vi "set_context.vi"(8 "error in (no error)":errorcluster, 9 "remote address":string, 10 "remote port":u16, 11 "WebSocket Queue Logger in":refnum<class "WebSocket Queue Logger.lvclass">) -> (0 "error out":errorcluster, 3 "WebSocket Queue Logger out":refnum<class "WebSocket Queue Logger.lvclass">)   [LabVIEW 2019, in "WebSocket Server Toolkit.lvlib" / "WebSocket Queue Logger.lvclass"]
uses:
  WebSocket Queue Logger.lvclass
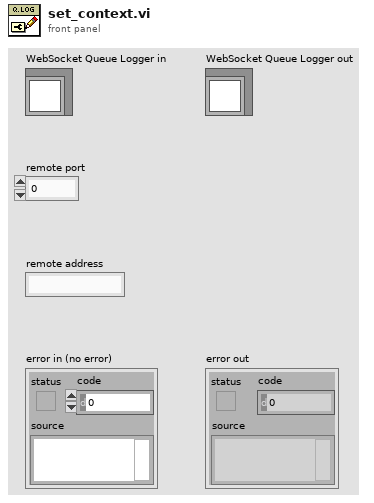
[diagram p1: front panel]
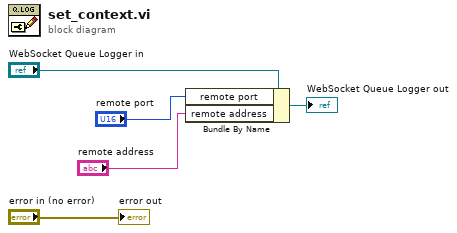
[diagram p0: block diagram]
diagram:
  n1 = Bundle By Name(cluster="WebSocket Queue Logger in", "remote port"="remote port", "remote address"="remote address") -> (→"WebSocket Queue Logger out":refnum<class "WebSocket Queue Logger.lvclass">)
  "error out" <- "error in (no error)"
